vi "Extract Becker-Hickl Binary Setup Parameters.vi"(8 "Error In":errorcluster, 11 "B&H Setup String":string) -> (0 "Error Out":errorcluster)   [LabVIEW 2021, in "Becker-Hickl Files.lvlib"]
uses:
  Becker-Hickl Files.lvlib
  Becker-Hickl Binary Setup Parameters.ctl
  Becker-Hickl Read Single I16.vi
  Becker-Hickl Read Single U32.vi
  Becker-Hickl Read Single U16.vi
panel:
  out "Binary Setup Length":i16
  out "Binary Setup":T1
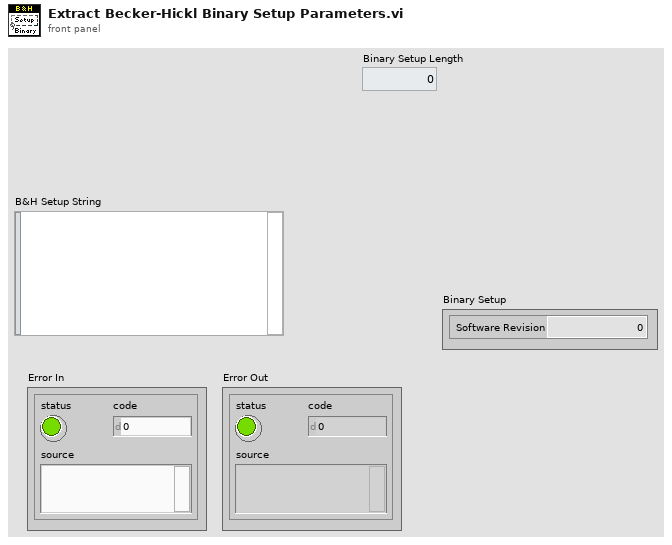
[diagram p1: front panel]
types:
  T1 = typedef "Becker-Hickl Files.lvlib/Becker-Hickl Binary Setup Parameters.ctl" = cluster{"Software Revision":u32}
  T2 = enum16{"soft_ref", "para_length", "reserved1", "reserved2"}
  T3 = enum16{"FCS_old_offs", "FCS_old_size", "gr1_offs", "gr1_size", "FCS_offs", "FCS_size", "FIDA_offs", "FIDA_size", "FILDA_offs", "FILDA_size", "gr2_offs", "gr_no", "hst_no", "hst_offs", "GVD_offs", "GVD_size", "FIT_offs", "FIT_size", "extdev_offs", "extdev_size", "reserve2", "reserve3"}
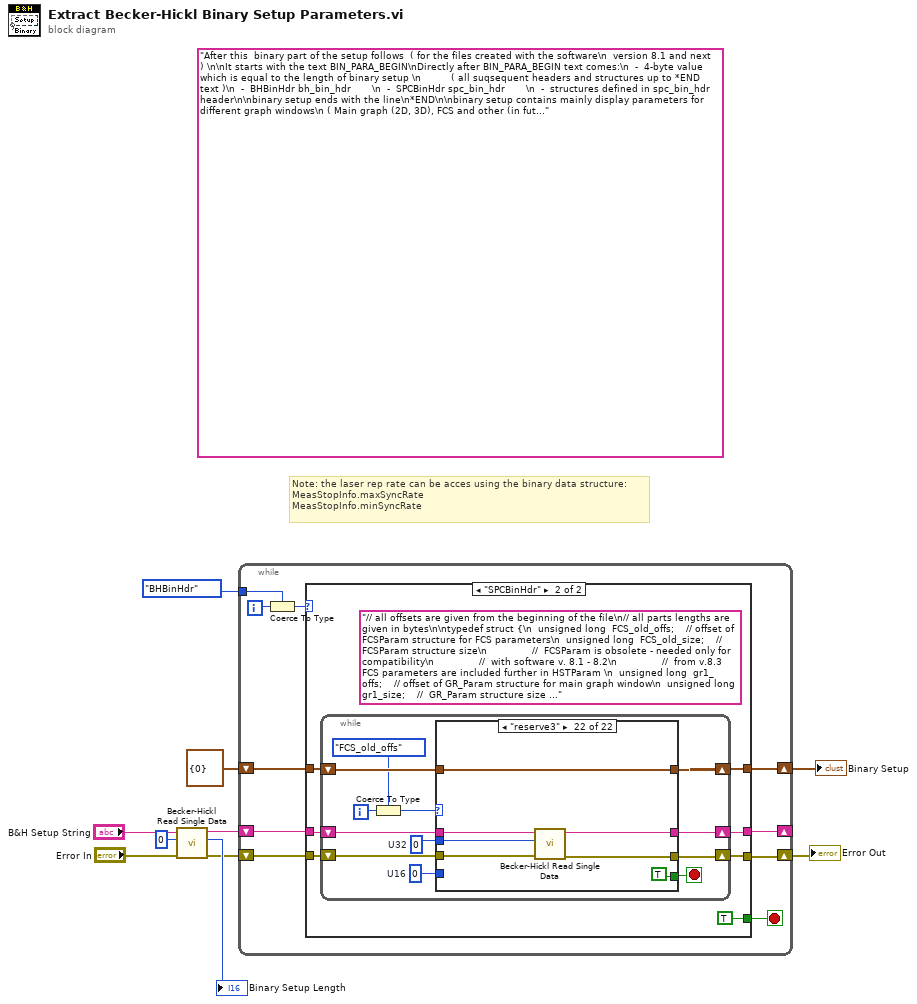
[diagram p0: block diagram]
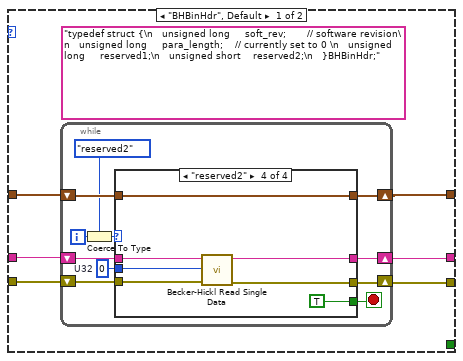
[diagram p2: hidden frame]
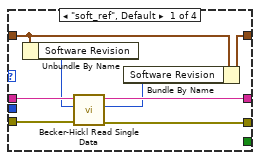
[diagram p3: hidden frame]
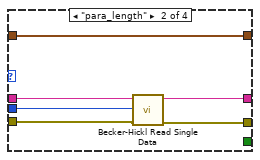
[diagram p4: hidden frame]
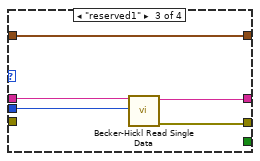
[diagram p5: hidden frame]
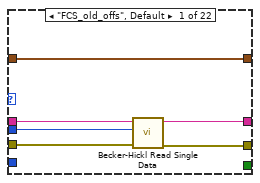
[diagram p6: hidden frame]
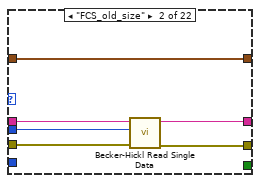
[diagram p7: hidden frame]
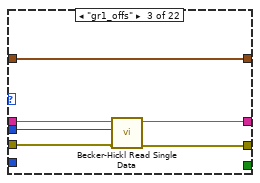
[diagram p8: hidden frame]
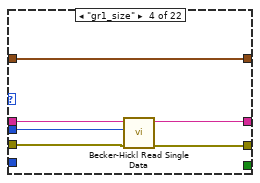
[diagram p9: hidden frame]
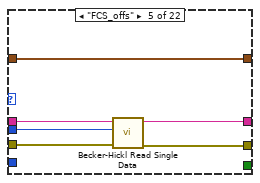
[diagram p10: hidden frame]
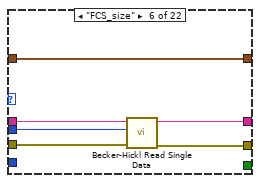
[diagram p11: hidden frame]
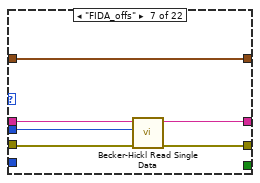
[diagram p12: hidden frame]
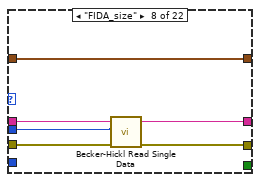
[diagram p13: hidden frame]
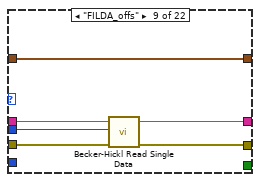
[diagram p14: hidden frame]
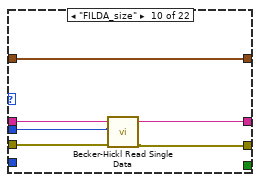
[diagram p15: hidden frame]
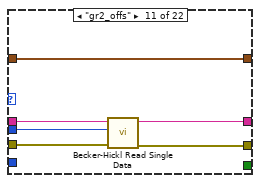
[diagram p16: hidden frame]
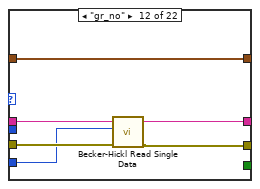
[diagram p17: hidden frame]
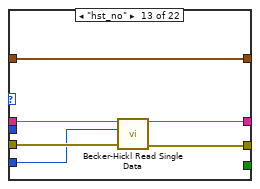
[diagram p18: hidden frame]
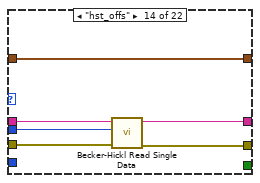
[diagram p19: hidden frame]
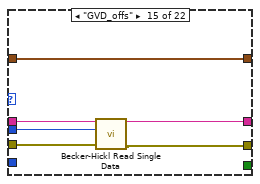
[diagram p20: hidden frame]
diagram:
  (unwired) "After this  binary part of the setup follows  ( for the files created with the software\n  version 8.1 and next ) \n\nIt starts with the text BIN_PARA_BEGIN\nDirectly after BIN_PARA_BEGIN text comes:\n  -  4-byte value which is equal to the length of binary setup \n          ( all suqsequent headers and structures up to *END text )\n  -  BHBinHdr bh_bin_hdr       \n  -  SPCBinHdr spc_bin_hdr       \n  -  structures defined in spc_bin_hdr header\n\nbinary setup ends with the line\n*END\n\nbinary setup contains mainly display parameters for different graph windows\n ( Main graph (2D, 3D), FCS and other (in future) ), \n which are used by the main software to restore display parameters\n   of the specific windows\n DI_ parameters in ASCII part of the setup are now obsolete and are present\n for compatibility reason only\n*/\n\ntypedef struct {\n   unsigned long     soft_rev;       // software revision\n   unsigned long     para_length;    // currently set to 0 \n   unsigned long     reserved1;\n   unsigned short    reserved2;\n   }BHBinHdr;\n\n\n// all offsets are given from the beginning of the file\n// all parts lengths are given in bytes\n\ntypedef struct {\n  unsigned long  FCS_old_offs;    // offset of FCSParam structure for FCS parameters\n  unsigned long  FCS_old_size;    //  FCSParam structure size\n               //  FCSParam is obsolete - needed only for compatibility\n               //  with software v. 8.1 - 8.2\n               //  from v.8.3 FCS parameters are included further in HSTParam \n  unsigned long  gr1_offs;    // offset of GR_Param structure for main graph window\n  unsigned long  gr1_size;    //  GR_Param structure size                       \n  unsigned long  FCS_offs;    // offset of HSTParam structure for FCS parameters\n  unsigned long  FCS_size;    //  HSTParam structure size\n  unsigned long  FIDA_offs;   // offset of HSTParam structure for FIDA window parameters\n  unsigned long  FIDA_size;   //  HSTParam structure size \n  unsigned long  FILDA_offs;  // offset of HSTParam structure for FILDA window parameters\n  unsigned long  FILDA_size;  //  HSTParam structure size\n  unsigned long  gr2_offs;    // offset of GR_Param structure for the 1st additional graph\n  unsigned short gr_no;       // number of additional GR_Param structures, ( size = gr1_size )\n  unsigned short hst_no;      // number of additional HSTParam structures, ( size = FCS_size )\n  unsigned long  hst_offs;    // offset of the 1st additional HSTParam structure\n  unsigned long  GVD_offs;    // offset of GVDParam structure for GVD-120 parameters \n  unsigned short GVD_size;    //  GVDParam structure size\n  unsigned short FIT_offs;    // offset of FITSetup structure for FIT parameters\n  unsigned short FIT_size;    //  FITSetup structure size\n  unsigned short extdev_offs;  // offset of external devices setup structures\n  unsigned short extdev_size;  //  size of external devices setup structures\n  unsigned short reserve2;\n  unsigned long  reserve3;\n  }SPCBinHdr;\n\n/*\nSPCBinHdr header includes offsets of GR_Param structure for the main display window\n  and HSTParam structures for FCS, FIDA and FILDA windows.\nAnother GR_Param structures can be included if additional 3D display windows were \n  opened\nAnother HSTParam structures can be included if additional histograms windows were \n  opened ( e.g. MCS (Macro Time) histogram )\nGVDParam structure contains parameters of GVD-120 module which controls BH Galvano Scanner.\nFITParam structure contains start values of FCS fitting parameters   \nOther fields will be used in future software versions\nFCS, FIDA, FILDA, MCS windows parameters are defined below in HSTParam structure\nThe structure contains attributes of histogram display windows,\n  which can be visible in FIFO mode\n*/\n\ntypedef struct {\n  int   top;\n  int   left;\n  int   height;\n  int   width;\n  int   flags;  // 0x1 - visible\n  }BHPanelAttr;\n\n\n\ntypedef union \n{\n  int             i;\n  unsigned int    u;\n  int             b;\n  short           h;\n  unsigned short  g;\n  long            l;\n  unsigned long   m;\n  float           f;\n  double          d;\n  char            c;\n} DparVal;\n\n\n\n  \n  \ntypedef struct            \n{\n  DparVal maxcnt;     //  DI_MAXCNT    \n  DparVal lbline;     //  DI_LBLINE  \n  DparVal bline;      //  DI_BLINE     \n  int  scale;         //  DI_SCALE   \n  int  grid;          //  DI_GRID  X : bit1, bit3 minor/ Y : bit2, bit 4 minor/ bit0 = X+Y\n  int  plot_style;    //  DI_TRACE     \n  int  point_style;   //  DI_PSTYLE    \n  int  line_style;    //  set to 0    \n  int  point_freq;    //  DI_PFREQ   \n  int  resize;        //  0 - not set, 1- Full size, 2 - Proportional, 3- other\n  int   grid_color;   //  DI_GCOL_F\n  int   bkg_color;    //  DI_GCOL_B\n  int   d2_mode;      //  DI_2DDIS\n  short reverse;      //  DI_XREV - bit 0, DI_YREV - bit 1                          \n  short ascale;       //  autoscale for 2D\n  DparVal xlow;          \n  DparVal xhigh;          \n  int  xscale;        //  Xscale log = 1\n  DparVal yhilim;     // high limit for y scale  \n} Disp2DAttr;\n\n\n\n\ntypedef struct  {    // obsolete, needed only for compatibility with software v. 8.1 - 8.2\n  int      view_decay;      \n  int      view_fcs;   \n  float    cortime; // correlation time [ms] \n  BHPanelAttr  pnl_attr; \n  Disp2DAttr   d2para;\n  }FCSParam;\n\n\n// Histogram traces parameters ( FCS, FIDA, FILDA, MCS )\ntypedef struct  {\n  short    active;         // (0)1 - (not) active   \n  short    module;\n  short    curve;          // routing channel no \n  short    cross_curve;    // cross correlation channel number for FCS\n                      //    ( when = curve and module = cross_module -  auto FCS )\n  short    cross_module;   // cross correlation module number for FCS\n  int      color;          // trace color\n  int      points;         // number of points in trace \n  }HSTtrace;  //\n\n\n\n#define MAX_NO_OF_TRACES  8\n\ntypedef struct{        // structure for FCS, FIDA and FILDA histogram windows\n  int              active;   // window visible, histogram is calculated\n  unsigned short   hst_type; // additional histogram parameters\n                    // for FCS:  0 - linear FCS with log binning ( 100 bins/log )\n                              // when bit 15 = 1 ( 0x8000 ) - Multi-Tau FCS \n                              //           where bits 14-0 = ktau parameter\n  short          reserve;   \n  float          time;     // in [ms], correlation time for FCS, \n                           // period time for FIDA, FILDA, time per point for MT\n  BHPanelAttr    pnl_attr; \n  Disp2DAttr     d2para;\n  HSTtrace       htrace[MAX_NO_OF_TRACES];\n  }HSTParam;\n\n\n\n#define MAX_NO_OF_COLORS   11 // max value for DI_COL_NO\n\ntypedef struct            \n{\n  int   offsx;             //  DI_3DOFFX - offset X for 3D display \n  int   offsy;             //  DI_3DOFFY - offset Y for 3D display         \n  int   inclination;       //  DI_3DINCX - inclination X for 3D display    \n  int   body_color;        //  DI_BOD_C\n  int   curve_color;       //  DI_3DCOL\n  int   d3_mode;           //  DI_3DMODE\n  int   ywin;              //  DI_YWIN  \n  int   xwin;              //  DI_XWIN  \n  int   twin;              //  DI_TWIN  \n  int   sywin;             //  DI_SYWIN  \n  int   sxwin;             //  DI_SXWIN  \n  int   d3_style;          //  DI_3DSTYL\n  int   interpolate;       //  DI_INTCOL- bit 0, DI_INTPIX - bit 1\n  int   col_no;            //  DI_COL_NO\n  int   color[MAX_NO_OF_COLORS];   // 0 - DI_COLMIN, 1 - DI_COLMAX, 2..5 - DI_COL2-5,\n                           // 6 - 10 are stored in BIN_SETUP\n  int   col_hi;            //  DI_HICOL\n  int   detail;            //  DI_DETAIL  \n  int   ascale;            //  DI_ASCALE  \n  int   lcol_no;           //  DI_COL_NO  for log scale\n} Disp3DAttr;\n\n\n\ntypedef struct _Interval {\n    unsigned int    from;\n    unsigned int    to;\n    }Interval;\n\n\n\ntypedef struct _Trace3d {\n  short    log_scale;       /*  display type 0- linear , 1- logarithmic  */\n  short    offsx;           /*  display offset X  - parameter DI_3DOFFX  */\n  short    offsy;           /*  display offset Y  - parameter DI_3DOFFY  */\n  double   inclination;     /*  display inclination- parameter DI_3DINCX  */\n  short    mode;            /*  display mode  - parameter DI_3DMODE  */\n  unsigned int    page;            /*  page number in SPC memory */\n  unsigned int    no_of_curves;    /*  number of curves  */\n  unsigned int    no_of_disp_curves;    /*  number of displayed curves */\n  unsigned int    no_of_points;    /*  number of points  */\n  short    resolution; \n  Interval * win;            /*  pointer to  window interval - depending on\n                                   display mode = DI_XWIN,DI_YWIN,DI_TWIN */\n  Interval * win_y;          /*  pointer to Y window interval - for f(t,x,y,param) */\n  unsigned short  first_disp_point; /*  number of first displayed point on curves  */\n  unsigned short  last_disp_point;  /*  number of last displayed point on curves  */\n  unsigned int    first_disp_curve; /*  number of first displayed curve  */\n  unsigned int    last_disp_curve;  /*  number of last displayed curve  */\n  short    reduction;        /*  display reduction ratio  */\n  int      color;            /*  colors of curves  (DIS_3DCOL converted ) */\n  int      body_color;       /*  color of the body (DIS_BOD_C converted ) */\n  double   curve1_xpos;      /*  x position on the graph of the first curve */\n  double   curve1_ypos;      /*  y position on the graph of the first curve */\n  double   xinc;             /*  x increment */\n  double   yinc;             /*  y increment */\n  double   ygain;            /*  y gain */\n  short    no;               /*  3d trace no */\n  short    sreserve;         /*  for future use */\n  unsigned long    reserve;  /*  for future use */\n  long     low_offset;       /*  DI_BLINE */\n  long     max_count;        /*  DI_MAXCNT */\n  Interval * swin;           /*  pointer to ScanX(Y) window interval -  depending on\n                                 display mode = DI_XWIN,DI_YWIN,DI_TWIN */\n  Interval * swin_y;         /*  pointer to ScanY window interval  */\n  long no_of_blocks;         /*  for get3Dcurve */\n  } Trace3d;\n\n\n\ntypedef struct  {\n  short               active;      \n  unsigned short      tr3d_module; // mod_no for 3D trace, missing in Trace3d structure\n  unsigned short      mem_bank;      \n  unsigned short      reserved2;      \n  double              dreserved1;\n  double              dreserved2;\n  BHPanelAttr         pnl_attr; \n  Disp2DAttr          d2para;    // Disp2DAttr for modes with 2D display  \n  Disp3DAttr          d3para;    // additional parameters for 3D display  \n  Disp2DAttr          d23para;   // Disp2DAttr for modes with 3D display  \n  Trace3d             tr3d;      // 3D trace parameters structure                                      \n  Disp2DAttr          d21para;   // Disp2DAttr for modes with 2D display and 32-bit range\n                                 //      ( fifo modes & 2D Block Display )\n  }GR_Param;                     // Main Graph window parameters\n\n\n"
  # "Note: the laser rep rate can be acces using the binary data structure:\nMeasStopInfo.maxSyncRate\nMeasStopInfo.minSyncRate"
  n1 = call-poly "Becker-Hickl Read Single Data.vi"("Error In"="Error In", "Default"=i16 0, "Bytes in"="B&H Setup String") -> ("Error Out"=w3:errorcluster, "I16"=→"Binary Setup Length":i16, "Bytes out"=w6:string)  [unwired: 6 in]
  n2 = while {
    tunnel: enum16{"BHBinHdr", "SPCBinHdr"}."BHBinHdr" -> [w18]
    shift-right: [w16] -> w7
    shift-left: T1 {"Software Revision"=0} ("Binary Setup") -> [w17]
    shift-right: [w14] -> _
    shift-left: w6 -> [w15]
    shift-right: [w11] -> w1
    shift-left: w3 -> [w12]
    i -> [w20]
    stop <- w13 stop-if-true
    n3 = Coerce To Type(0:w20, 1:w18) -> (2:w19:enum16{"BHBinHdr", "SPCBinHdr"})
    n4 = case shown="\"SPCBinHdr\"" w19 {
      tunnel: w17 -> [w26 w70]
      tunnel: [w25 w69] -> w16
      tunnel: w15 -> [w24 w68]
      tunnel: [w23 w67] -> w14
      tunnel: [_ TRUE] -> w13
      tunnel: w12 -> [w22 w65]
      tunnel: [w21 w64] -> w11
      frame "BHBinHdr", Default {
        (unwired) "typedef struct {\n   unsigned long     soft_rev;       // software revision\n   unsigned long     para_length;    // currently set to 0 \n   unsigned long     reserved1;\n   unsigned short    reserved2;\n   }BHBinHdr;"
        n5 = while {
          shift-right: [w35] -> w23
          shift-left: w24 -> [w36]
          shift-right: [w32] -> w25
          shift-left: w26 -> [w33]
          shift-right: [w28] -> w21
          shift-left: w22 -> [w29]
          i -> [w37]
          stop <- w34 stop-if-true
          w27 = u32 0  # U32
          n6 = Coerce To Type(0:w37, 1:T2."reserved2") -> (2:w31:T2)
          n7 = case shown="\"reserved2\"" w31 {
            tunnel: w36 -> [w44 w50 w55 w61]
            tunnel: [w43 w49 w54 w60] -> w35
            tunnel: [_ _ _ TRUE] -> w34
            tunnel: w33 -> [w39 w51 w56 w62]
            tunnel: [w45 w51 w56 w62] -> w32
            tunnel: w29 -> [w41 w48 _ w59]
            tunnel: [w40 w46 w52 w58] -> w28
            tunnel: w27 -> [_ w47 w53 w57]
            frame "soft_ref", Default {
              # "soft_rev"
              n8 = Unbundle By Name(w39) -> ("Software Revision"=w38:u32)
              n9 = call-poly "Becker-Hickl Read Single Data.vi"("Error In"=w41, "Default"=w38, "Bytes in"=w44) -> ("Error Out"=w40:errorcluster, "U32"=w42:u32, "Bytes out"=w43:string)  [unwired: 6 in]
              n10 = Bundle By Name(cluster=w39, "Software Revision"=w42) -> (w45:T1)
            }
            frame "para_length" {
              # "para_length"
              n11 = call-poly "Becker-Hickl Read Single Data.vi"("Error In"=w48, "Default"=w47, "Bytes in"=w50) -> ("Error Out"=w46:errorcluster, "Bytes out"=w49:string)  [unwired: 6 in, 1 out]
            }
            frame "reserved1" {
              # "reserved1"
              n12 = call-poly "Becker-Hickl Read Single Data.vi"("Default"=w53, "Bytes in"=w55) -> ("Error Out"=w52:errorcluster, "Bytes out"=w54:string)  [unwired: 7 in, 1 out]
            }
            frame "reserved2" {
              # "reserved2"
              n13 = call-poly "Becker-Hickl Read Single Data.vi"("Error In"=w59, "Default"=w57, "Bytes in"=w61) -> ("Error Out"=w58:errorcluster, "Bytes out"=w60:string)  [unwired: 6 in, 1 out]
            }
          }
        }
      }
      frame "SPCBinHdr" {
        (unwired) "// all offsets are given from the beginning of the file\n// all parts lengths are given in bytes\n\ntypedef struct {\n  unsigned long  FCS_old_offs;    // offset of FCSParam structure for FCS parameters\n  unsigned long  FCS_old_size;    //  FCSParam structure size\n               //  FCSParam is obsolete - needed only for compatibility\n               //  with software v. 8.1 - 8.2\n               //  from v.8.3 FCS parameters are included further in HSTParam \n  unsigned long  gr1_offs;    // offset of GR_Param structure for main graph window\n  unsigned long  gr1_size;    //  GR_Param structure size                       \n  unsigned long  FCS_offs;    // offset of HSTParam structure for FCS parameters\n  unsigned long  FCS_size;    //  HSTParam structure size\n  unsigned long  FIDA_offs;   // offset of HSTParam structure for FIDA window parameters\n  unsigned long  FIDA_size;   //  HSTParam structure size \n  unsigned long  FILDA_offs;  // offset of HSTParam structure for FILDA window parameters\n  unsigned long  FILDA_size;  //  HSTParam structure size\n  unsigned long  gr2_offs;    // offset of GR_Param structure for the 1st additional graph\n  unsigned short gr_no;       // number of additional GR_Param structures, ( size = gr1_size )\n  unsigned short hst_no;      // number of additional HSTParam structures, ( size = FCS_size )\n  unsigned long  hst_offs;    // offset of the 1st additional HSTParam structure\n  unsigned long  GVD_offs;    // offset of GVDParam structure for GVD-120 parameters \n  unsigned short GVD_size;    //  GVDParam structure size\n  unsigned short FIT_offs;    // offset of FITSetup structure for FIT parameters\n  unsigned short FIT_size;    //  FITSetup structure size\n  unsigned short extdev_offs;  // offset of external devices setup structures\n  unsigned short extdev_size;  //  size of external devices setup structures\n  unsigned short reserve2;\n  unsigned long  reserve3;\n  }SPCBinHdr;"
        n14 = while {
          shift-right: [w80] -> w67
          shift-left: w68 -> [w81]
          shift-right: [w78] -> w69
          shift-left: w70 -> [w79]
          shift-right: [w73] -> w64
          shift-left: w65 -> [w74]
          i -> [w82]
          stop <- w75 stop-if-true
          w71 = u16 0  # U16
          w72 = u32 0  # U32
          n15 = Coerce To Type(0:w82, 1:T3."FCS_old_offs") -> (2:w77:T3)
          n16 = case shown="\"reserve3\"" w77 {
            tunnel: w81 -> [w87 w93 w99 w105 w111 w117 w123 w129 w135 w141 w147 w153 w159 w165 w171 w177 w183 w189 w195 w201 w207 w214]
            tunnel: [w86 w92 w98 w104 w110 w116 w122 w128 w134 w140 w146 w152 w158 w164 w170 w176 w182 w188 w194 w200 w206 w213] -> w80
            tunnel: [_ _ _ _ _ _ _ _ _ _ _ _ _ _ _ _ _ _ _ _ _ TRUE] -> w75
            tunnel: w79 -> [w88 w94 w100 w106 w112 w118 w124 w130 w136 w142 w148 w154 w160 w166 w172 w178 w184 w190 w196 w202 w208 w215]
            tunnel: [w88 w94 w100 w106 w112 w118 w124 w130 w136 w142 w148 w154 w160 w166 w172 w178 w184 w190 w196 w202 w208 w215] -> w78
            tunnel: w74 -> [w85 w90 w97 w102 w109 w115 w121 w127 w133 w139 w145 w151 w157 w163 w169 w175 w181 w187 w193 w199 w205 w211]
            tunnel: [w84 w89 w96 w101 w107 w113 w120 w126 w131 w138 w144 w150 w156 w162 w168 w174 w180 w186 w192 w198 w204 w210] -> w73
            tunnel: w72 -> [w83 w91 w95 w103 w108 w114 w119 w125 w132 w137 w143 _ _ w161 w167 _ _ _ _ _ _ w209]
            tunnel: w71 -> [_ _ _ _ _ _ _ _ _ _ _ w149 w155 _ _ w173 w179 w185 w191 w197 w203 _]
            frame "FCS_old_offs", Default {
              n17 = call-poly "Becker-Hickl Read Single Data.vi"("Error In"=w85, "Default"=w83, "Bytes in"=w87) -> ("Error Out"=w84:errorcluster, "Bytes out"=w86:string)  [unwired: 6 in, 1 out]
            }
            frame "FCS_old_size" {
              n18 = call-poly "Becker-Hickl Read Single Data.vi"("Error In"=w90, "Default"=w91, "Bytes in"=w93) -> ("Error Out"=w89:errorcluster, "Bytes out"=w92:string)  [unwired: 6 in, 1 out]
            }
            frame "gr1_offs" {
              n19 = call-poly "Becker-Hickl Read Single Data.vi"("Error In"=w97, "Default"=w95, "Bytes in"=w99) -> ("Error Out"=w96:errorcluster, "Bytes out"=w98:string)  [unwired: 6 in, 1 out]
            }
            frame "gr1_size" {
              n20 = call-poly "Becker-Hickl Read Single Data.vi"("Error In"=w102, "Default"=w103, "Bytes in"=w105) -> ("Error Out"=w101:errorcluster, "Bytes out"=w104:string)  [unwired: 6 in, 1 out]
            }
            frame "FCS_offs" {
              n21 = call-poly "Becker-Hickl Read Single Data.vi"("Error In"=w109, "Default"=w108, "Bytes in"=w111) -> ("Error Out"=w107:errorcluster, "Bytes out"=w110:string)  [unwired: 6 in, 1 out]
            }
            frame "FCS_size" {
              n22 = call-poly "Becker-Hickl Read Single Data.vi"("Error In"=w115, "Default"=w114, "Bytes in"=w117) -> ("Error Out"=w113:errorcluster, "Bytes out"=w116:string)  [unwired: 6 in, 1 out]
            }
            frame "FIDA_offs" {
              n23 = call-poly "Becker-Hickl Read Single Data.vi"("Error In"=w121, "Default"=w119, "Bytes in"=w123) -> ("Error Out"=w120:errorcluster, "Bytes out"=w122:string)  [unwired: 6 in, 1 out]
            }
            frame "FIDA_size" {
              n24 = call-poly "Becker-Hickl Read Single Data.vi"("Error In"=w127, "Default"=w125, "Bytes in"=w129) -> ("Error Out"=w126:errorcluster, "Bytes out"=w128:string)  [unwired: 6 in, 1 out]
            }
            frame "FILDA_offs" {
              n25 = call-poly "Becker-Hickl Read Single Data.vi"("Error In"=w133, "Default"=w132, "Bytes in"=w135) -> ("Error Out"=w131:errorcluster, "Bytes out"=w134:string)  [unwired: 6 in, 1 out]
            }
            frame "FILDA_size" {
              n26 = call-poly "Becker-Hickl Read Single Data.vi"("Error In"=w139, "Default"=w137, "Bytes in"=w141) -> ("Error Out"=w138:errorcluster, "Bytes out"=w140:string)  [unwired: 6 in, 1 out]
            }
            frame "gr2_offs" {
              n27 = call-poly "Becker-Hickl Read Single Data.vi"("Error In"=w145, "Default"=w143, "Bytes in"=w147) -> ("Error Out"=w144:errorcluster, "Bytes out"=w146:string)  [unwired: 6 in, 1 out]
            }
            frame "gr_no" {
              n28 = call-poly "Becker-Hickl Read Single Data.vi"("Error In"=w151, "Default"=w149, "Bytes in"=w153) -> ("Error Out"=w150:errorcluster, "Bytes out"=w152:string)  [unwired: 6 in, 1 out]
            }
            frame "hst_no" {
              n29 = call-poly "Becker-Hickl Read Single Data.vi"("Error In"=w157, "Default"=w155, "Bytes in"=w159) -> ("Error Out"=w156:errorcluster, "Bytes out"=w158:string)  [unwired: 6 in, 1 out]
            }
            frame "hst_offs" {
              n30 = call-poly "Becker-Hickl Read Single Data.vi"("Error In"=w163, "Default"=w161, "Bytes in"=w165) -> ("Error Out"=w162:errorcluster, "Bytes out"=w164:string)  [unwired: 6 in, 1 out]
            }
            frame "GVD_offs" {
              n31 = call-poly "Becker-Hickl Read Single Data.vi"("Error In"=w169, "Default"=w167, "Bytes in"=w171) -> ("Error Out"=w168:errorcluster, "Bytes out"=w170:string)  [unwired: 6 in, 1 out]
            }
            frame "GVD_size" {
              n32 = call-poly "Becker-Hickl Read Single Data.vi"("Error In"=w175, "Default"=w173, "Bytes in"=w177) -> ("Error Out"=w174:errorcluster, "Bytes out"=w176:string)  [unwired: 6 in, 1 out]
            }
            frame "FIT_offs" {
              n33 = call-poly "Becker-Hickl Read Single Data.vi"("Error In"=w181, "Default"=w179, "Bytes in"=w183) -> ("Error Out"=w180:errorcluster, "Bytes out"=w182:string)  [unwired: 6 in, 1 out]
            }
            frame "FIT_size" {
              n34 = call-poly "Becker-Hickl Read Single Data.vi"("Error In"=w187, "Default"=w185, "Bytes in"=w189) -> ("Error Out"=w186:errorcluster, "Bytes out"=w188:string)  [unwired: 6 in, 1 out]
            }
            frame "extdev_offs" {
              n35 = call-poly "Becker-Hickl Read Single Data.vi"("Error In"=w193, "Default"=w191, "Bytes in"=w195) -> ("Error Out"=w192:errorcluster, "Bytes out"=w194:string)  [unwired: 6 in, 1 out]
            }
            frame "extdev_size" {
              n36 = call-poly "Becker-Hickl Read Single Data.vi"("Error In"=w199, "Default"=w197, "Bytes in"=w201) -> ("Error Out"=w198:errorcluster, "Bytes out"=w200:string)  [unwired: 6 in, 1 out]
            }
            frame "reserve2" {
              n37 = call-poly "Becker-Hickl Read Single Data.vi"("Error In"=w205, "Default"=w203, "Bytes in"=w207) -> ("Error Out"=w204:errorcluster, "Bytes out"=w206:string)  [unwired: 6 in, 1 out]
            }
            frame "reserve3" {
              n38 = call-poly "Becker-Hickl Read Single Data.vi"("Error In"=w211, "Default"=w209, "Bytes in"=w214) -> ("Error Out"=w210:errorcluster, "Bytes out"=w213:string)  [unwired: 6 in, 1 out]
            }
          }
        }
      }
    }
  }
  "Error Out" <- w1
  "Binary Setup" <- w7
